vi "Rank Transformation.vi"(11 "x":dbl[](array[numeric]) format="%.2f") -> (1 "tsum - measure of ties":dbl format="%#.6g", 3 "rank order x":dbl[](array[numeric]) format="%.2f")   [LabVIEW 2020, in "NI_Gmath.lvlib"]
doc: "Finds the rank order of each element in the <B>x</B> input and returns the order of each element in the <B>rank order x</B> output. For all tied rank values, the mean rank replaces the rank returned."
uses:
  <vilib>/gmath/NI_Gmath.lvlib
panel:
  # "Rank Transformation"
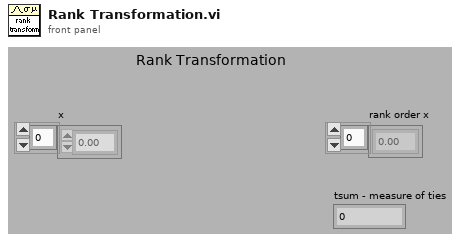
[diagram p1: front panel]
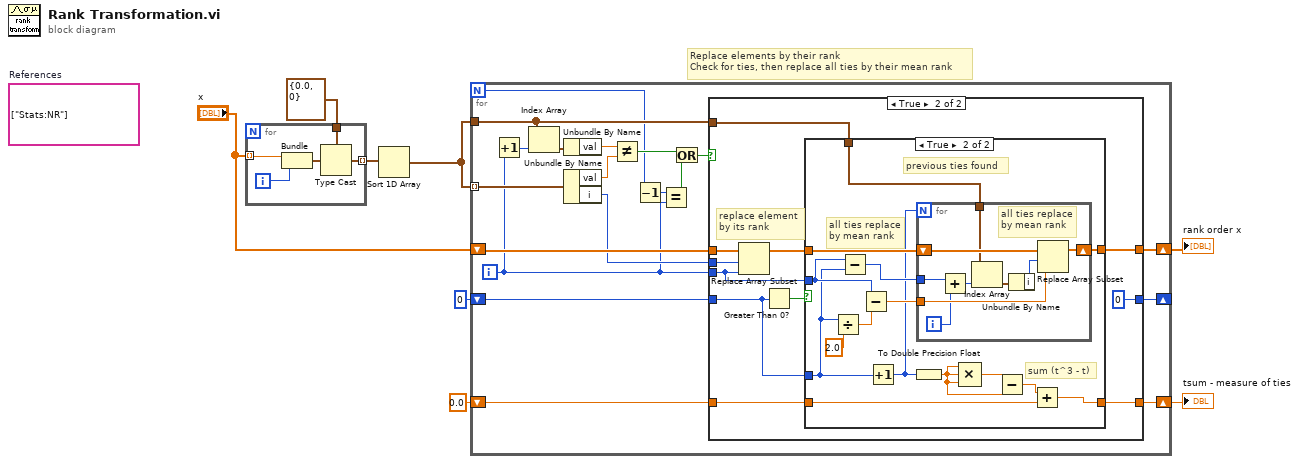
[diagram p0: block diagram]
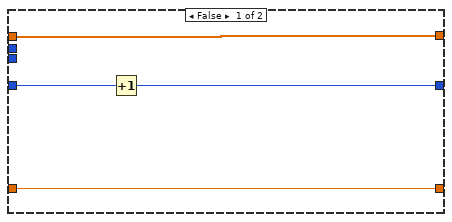
[diagram p2: hidden frame]
diagram:
  (unwired) string[] ["Stats:NR"]  # References
  # "Replace elements by their rank\nCheck for ties, then replace all ties by their mean rank"
  n1 = for {
    tunnel: "x" -> [w13] mode=indexing
    tunnel: [w11] -> w8 mode=indexing
    tunnel: cluster{"val":dbl, "i":i32} {"val"=0.0, "i"=0} -> [w10]
    i -> [w9]
    n2 = Bundle("Numeric"=w13, w9) -> (w12:cluster{"Numeric":dbl, i32})  [unwired: 1 in]
    n3 = Type Cast(type=w10, x=w12) -> (*(type *) &x=w11:cluster{"val":dbl, "i":i32})
  }
  n4 = Sort 1D Array(array=w8) -> (sorted array=w4:cluster{"val":dbl, "i":i32}[])
  n5 = for {
    N -> [w20]
    tunnel: w4 -> [w32] mode=indexing
    shift-right: [w29] -> w5
    shift-left: "x" -> [w31]
    tunnel: w4 -> [w23]
    shift-right: [w24] -> _
    shift-left: 0 -> [w25]
    shift-right: [w15] -> w2
    shift-left: 0.0 -> [w16]
    i -> [w18]
    n6 = Increment(x=w18) -> (x+1=w28:i32)
    n7 = Index Array(array=w23, index=w28) -> (element=w27:cluster{"val":dbl, "i":i32})
    n8 = Unbundle By Name(w27) -> ("val"=w26:dbl)
    n9 = Unbundle By Name(w32) -> ("val"=w14:dbl, "i"=w30:i32)
    n10 = Not Equal?(x=w26, y=w14) -> (x != y?=w21:bool)
    n11 = Decrement(x=w20) -> (x-1=w19:i32)
    n12 = Equal?(x=w19, y=w18) -> (x = y?=w17:bool)
    n13 = Or(x=w21, y=w17) -> (x .or. y?=w22:bool)
    n14 = case shown="True" w22 {
      tunnel: w31 -> [w36 w47]
      tunnel: w30 -> [_ w43]
      tunnel: [w36 w44] -> w29
      tunnel: w18 -> [_ w41]
      tunnel: w25 -> [w35 w40]
      tunnel: [w34 0] -> w24
      tunnel: w23 -> [_ w39]
      tunnel: w16 -> [w33 w38]
      tunnel: [w33 w37] -> w15
      frame False {
        n15 = Increment(x=w35) -> (x+1=w34:i32)
      }
      frame True {
        # "replace element\nby its rank"
        n16 = Replace Array Subset(array=w47, new element=w41, index=w43) -> (w45:dbl[])
        n17 = Greater Than 0?(x=w40) -> (x > 0?=w42:bool)
        n18 = case shown="True" w42 {
          tunnel: w45 -> [w49 w64]
          tunnel: [w49 w63] -> w44
          tunnel: w41 -> [_ w61]
          tunnel: w40 -> [_ w58]
          tunnel: w39 -> [_ w56]
          tunnel: w38 -> [w48 w51]
          tunnel: [w48 w50] -> w37
          frame False {
          }
          frame True {
            # "sum (t^3 - t)"
            # "all ties replace\nby mean rank"
            # "previous ties found"
            n19 = Divide(x=w58, y=2.0) -> (x/y=w60:dbl)
            n20 = Subtract(x=w61, y=w58) -> (x-y=w57:i32)
            n21 = Subtract(x=w61, y=w60) -> (x-y=w59:dbl)
            n22 = Increment(x=w58) -> (x+1=w55:i32)
            n23 = To Double Precision Float(number=w55) -> (double precision float=w53:dbl)
            n24 = for {
              N: w55 -> [_]
              tunnel: w59 -> [w71]
              shift-right: [w72] -> w63
              shift-left: w64 -> [w73]
              tunnel: w57 -> [w70]
              tunnel: w56 -> [w68]
              i -> [w69]
              # "all ties replace\nby mean rank"
              n25 = Add(x=w70, y=w69) -> (x+y=w67:i32)
              n26 = Index Array(array=w68, index=w67) -> (element=w66:cluster{"val":dbl, "i":i32})
              n27 = Unbundle By Name(w66) -> ("i"=w65:i32)
              n28 = Replace Array Subset(array=w73, new element=w71, index=w65) -> (w72:dbl[])
            }
            n29 = Compound Arithmetic op=MULTIPLY(w53, w53, w53) -> (w54:dbl)
            n30 = Subtract(x=w54, y=w53) -> (x-y=w52:dbl)
            n31 = Add(x=w52, y=w51) -> (x+y=w50:dbl)
          }
        }
      }
    }
  }
  "rank order x" <- w5
  "tsum - measure of ties" <- w2
